vi "conditionalENDOFFILEappend.vi"(8 "error in":errorcluster, 11 "refnum":refnum<file>) -> (0 "error out":errorcluster, 3 "refnum out":refnum<file>)   [LabVIEW 2019]
doc: "If the file has no ENDOFFILE keyword at the end of the file, append it."
panel:
  out "text":string
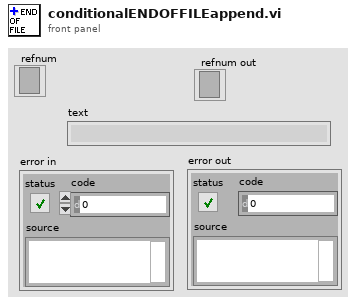
[diagram p1: front panel]
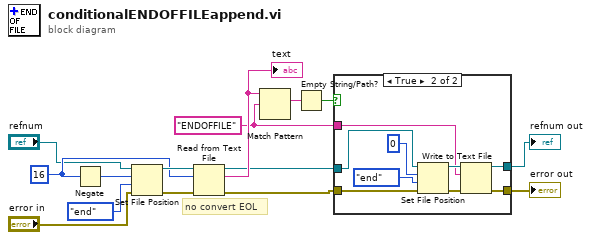
[diagram p0: block diagram]
diagram:
  w6 = "ENDOFFILE" ("text")
  w11 = i64 16 ("offset (in bytes) (0)")
  # "no convert EOL"
  n1 = Negate(x=w11) -> (-x=w12:i64)
  n2 = Set File Position(offset (in bytes) (0)=w12, refnum="refnum", from (0:start)=enum16{"start", "end", "current"}."end", error in="error in") -> (refnum out=w14:refnum<file>, error out=w13:errorcluster)
  n3 = Read from Text File(file (use dialog)=w14, count=w11, error in=w13) -> (refnum out=w7:refnum<file>, text=w10:string, error out=w5:errorcluster)  [unwired: 1 in, 1 out]
  "text" <- w10
  n4 = Match Pattern(string=w10, regular expression=w6) -> (match substring=w9:string)  [unwired: 1 in, 3 out]
  n5 = Empty String/Path?(string/path=w9) -> (empty?=w8:bool)
  n6 = case shown="True" w8 {
    tunnel: w7 -> [w17 w24]
    tunnel: w6 -> [_ w18]
    tunnel: [w17 w22] -> w2
    tunnel: [w16 w21] -> w1
    tunnel: w5 -> [w16 w19]
    frame False {
    }
    frame True {
      n7 = Set File Position(offset (in bytes) (0)=i64 0, refnum=w24, from (0:start)=enum16{"start", "end", "current"}."end", error in=w19) -> (refnum out=w23:refnum<file>, error out=w20:errorcluster)
      n8 = Write to Text File(file (use dialog)=w23, text=w18, error in=w20) -> (refnum out=w22:refnum<file>, error out=w21:errorcluster)  [unwired: 1 in, 1 out]
    }
  }
  "refnum out" <- w2
  "error out" <- w1
